vi "TCM_CmdStr.vi"(1 "TCM":T1 {"TCM指示转向灯开关状态" items=["默认", "转左", "转右", "无效"]}) -> (0 "CmdStr":string)   [LabVIEW 2013]
uses:
  TCM.ctl
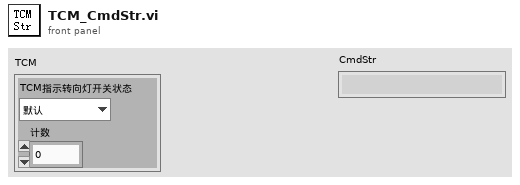
[diagram p1: front panel]
types:
  T1 = typedef "TCM.ctl" = cluster{"TCM指示转向灯开关状态":u16, "计数":u8}
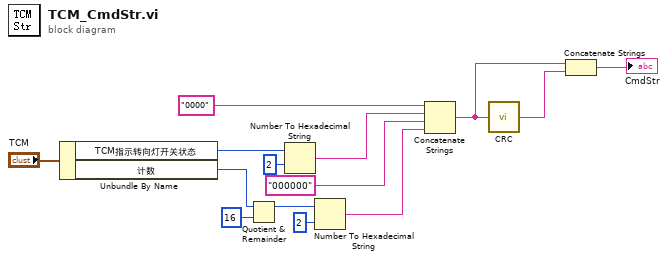
[diagram p0: block diagram]
diagram:
  n1 = Unbundle By Name("TCM") -> ("TCM指示转向灯开关状态"=w2:u16, "计数"=w1:u8)
  n2 = Quotient & Remainder(x=w1, y=u8 16) -> (x-y*floor(x/y)=w6:u8)  [unwired: 1 out]
  n3 = Number To Hexadecimal String(1:2, 2:w2) -> (0:w12:string)
  n4 = Number To Hexadecimal String(1:u8 2, 2:w6) -> (0:w5:string)
  n5 = Concatenate Strings("0000", w12, "000000", w5) -> (w9:string)
  n6 = call "CRC.vi"("StrIn"=w9) -> ("StrOut"=w10:string)
  n7 = Concatenate Strings(w9, w10) -> (→"CmdStr":string)
